vi "James.vi"(0 "Initial Case":enum16{"Theta", "Arc"}(ring), 5 "Drive Case":enum16{"FOD", "ROD"}(ring), 7 "Cyborg":dbl[](array[numeric]), 9 "Logitech":dbl[](array[numeric]), 11 "gyro":dbl format="%#_13g") -> (4 "A":dbl, 6 "B":dbl, 8 "R":dbl)   [LabVIEW 2014]
panel:
  in  "beta":dbl format="%#_13g"
  in  "alpha":dbl format="%#_13g"
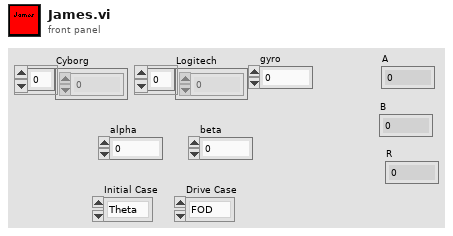
[diagram p1: front panel]
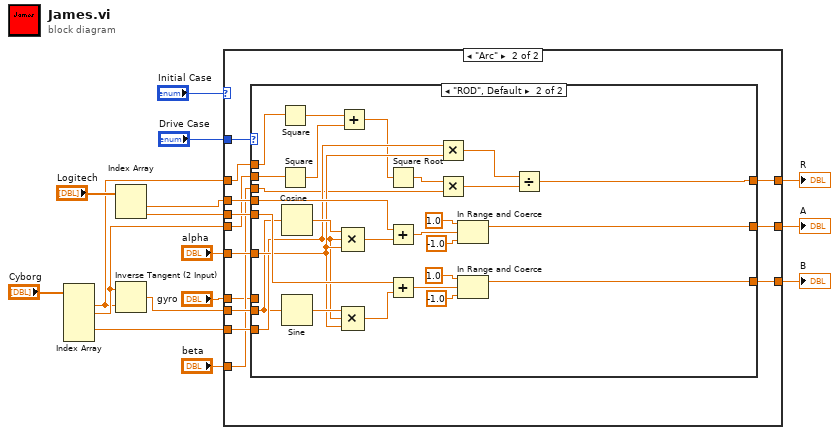
[diagram p0: block diagram]
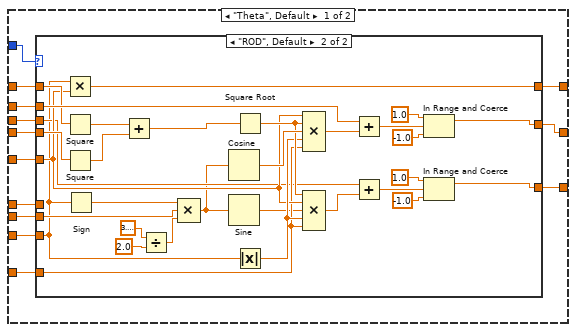
[diagram p2: hidden frame]
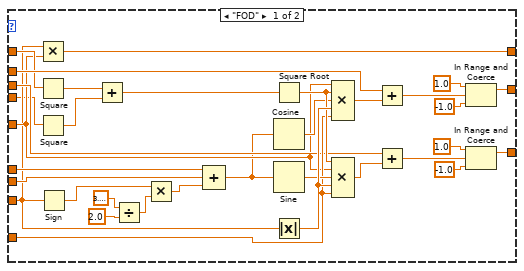
[diagram p3: hidden frame]
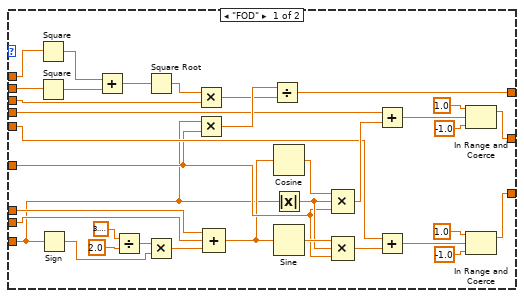
[diagram p4: hidden frame]
diagram:
  n1 = Index Array(array="Cyborg") -> (element #1=w5:dbl, element #2=w6:dbl, element #4=w11:dbl)  [unwired: 5 in, 2 out]
  n2 = Index Array(array="Logitech") -> (element #1=w9:dbl, element #2=w2:dbl)  [unwired: 2 in]
  n3 = Inverse Tangent (2 Input)(1:w5, 2:w6) -> (0:w8:dbl)
  n4 = case shown="\"Arc\"" "Initial Case" {
    tunnel: "Drive Case" -> [w29 w106]
    tunnel: w11 -> [w28 w104]
    tunnel: "alpha" -> [w27 w102]
    tunnel: [w26 w95] -> w13
    tunnel: w9 -> [w25 w105]
    tunnel: w8 -> [w24 w103]
    tunnel: "beta" -> [w23 w98]
    tunnel: w6 -> [w22 w96]
    tunnel: w5 -> [w21 w97]
    tunnel: [w20 w101] -> w4
    tunnel: [w19 w99] -> w3
    tunnel: w2 -> [w18 w100]
    tunnel: "gyro" -> [w17 w94]
    frame "Theta", Default {
      n5 = case shown="\"ROD\", Default" w29 {
        tunnel: w28 -> [w40 w72]
        tunnel: w27 -> [w49 w81]
        tunnel: [w37 w93] -> w26
        tunnel: w25 -> [w52 w92]
        tunnel: w24 -> [w43 w74]
        tunnel: w23 -> [w53 w80]
        tunnel: w22 -> [w39 w89]
        tunnel: w21 -> [w50 w88]
        tunnel: [w34 w64] -> w20
        tunnel: [w30 w69] -> w19
        tunnel: w18 -> [w51 w79]
        tunnel: w17 -> [w41 _]
        frame "FOD" {
          n6 = Multiply(x=w40, y=w49) -> (x*y=w37:dbl)
          n7 = Square(x=w50) -> (x^2=w57:dbl)
          n8 = Square(x=w39) -> (x^2=w56:dbl)
          n9 = Sign(1:w40) -> (0:w48:dbl)
          n10 = Add(x=w57, y=w56) -> (x+y=w58:dbl)
          n11 = Divide(x=3.141592653589793, y=2.0) -> (x/y=w45:dbl)
          n12 = Multiply(x=w48, y=w45) -> (x*y=w44:dbl)
          n13 = Compound Arithmetic op=ADD(w41, w43, w44) -> (w42:dbl)
          n14 = Square Root(x=w58) -> (sqrt(x)=w61:dbl)
          n15 = Cosine(x=w42) -> (cos(x)=w54:dbl)
          n16 = Sine(x=w42) -> (sin(x)=w59:dbl)
          n17 = Absolute Value(x=w40) -> (abs(x)=w62:dbl)
          n18 = Compound Arithmetic op=MULTIPLY(w49, w61, w54, w62, w53) -> (w55:dbl)
          n19 = Compound Arithmetic op=MULTIPLY(w61, w49, w59, w62, w53) -> (w60:dbl)
          n20 = Add(x=w52, y=w55) -> (x+y=w35:dbl)
          n21 = Add(x=w51, y=w60) -> (x+y=w31:dbl)
          n22 = In Range and Coerce(upper limit=1.0, x=w35, lower limit=-1.0) -> (coerced(x)=w34:dbl)  [unwired: 1 out]
          n23 = In Range and Coerce(upper limit=1.0, x=w31, lower limit=-1.0) -> (coerced(x)=w30:dbl)  [unwired: 1 out]
        }
        frame "ROD", Default {
          n24 = Multiply(x=w72, y=w81) -> (x*y=w93:dbl)
          n25 = Square(x=w88) -> (x^2=w86:dbl)
          n26 = Square(x=w89) -> (x^2=w87:dbl)
          n27 = Sign(1:w72) -> (0:w73:dbl)
          n28 = Add(x=w86, y=w87) -> (x+y=w85:dbl)
          n29 = Divide(x=3.141592653589793, y=2.0) -> (x/y=w77:dbl)
          n30 = Compound Arithmetic op=MULTIPLY(w73, w74, w77) -> (w71:dbl)
          n31 = Cosine(x=w71) -> (cos(x)=w91:dbl)
          n32 = Sine(x=w71) -> (sin(x)=w78:dbl)
          n33 = Square Root(x=w85) -> (sqrt(x)=w83:dbl)
          n34 = Absolute Value(x=w72) -> (abs(x)=w82:dbl)
          n35 = Compound Arithmetic op=MULTIPLY(w81, w83, w91, w82, w80) -> (w90:dbl)
          n36 = Compound Arithmetic op=MULTIPLY(w83, w81, w78, w82, w80) -> (w84:dbl)
          n37 = Add(x=w92, y=w90) -> (x+y=w65:dbl)
          n38 = Add(x=w79, y=w84) -> (x+y=w70:dbl)
          n39 = In Range and Coerce(upper limit=1.0, x=w65, lower limit=-1.0) -> (coerced(x)=w64:dbl)  [unwired: 1 out]
          n40 = In Range and Coerce(upper limit=1.0, x=w70, lower limit=-1.0) -> (coerced(x)=w69:dbl)  [unwired: 1 out]
        }
      }
    }
    frame "Arc" {
      n41 = case shown="\"ROD\", Default" w106 {
        tunnel: w105 -> [w130 w168]
        tunnel: w104 -> [w120 w160]
        tunnel: w103 -> [w122 w153]
        tunnel: w102 -> [w125 w161]
        tunnel: [w111 w142] -> w101
        tunnel: w100 -> [w129 w163]
        tunnel: [w107 w146] -> w99
        tunnel: w98 -> [w115 w159]
        tunnel: w97 -> [w128 w156]
        tunnel: w96 -> [w127 w154]
        tunnel: [w131 w151] -> w95
        tunnel: w94 -> [w124 _]
        frame "FOD" {
          n42 = Square(x=w128) -> (x^2=w135:dbl)
          n43 = Square(x=w127) -> (x^2=w134:dbl)
          n44 = Sign(1:w120) -> (0:w121:dbl)
          n45 = Add(x=w135, y=w134) -> (x+y=w132:dbl)
          n46 = Divide(x=3.141592653589793, y=2.0) -> (x/y=w117:dbl)
          n47 = Square Root(x=w132) -> (sqrt(x)=w136:dbl)
          n48 = Multiply(x=w117, y=w121) -> (x*y=w116:dbl)
          n49 = Multiply(x=w136, y=w115) -> (x*y=w133:dbl)
          n50 = Multiply(x=w120, y=w125) -> (x*y=w137:dbl)
          n51 = Compound Arithmetic op=ADD(w124, w122, w116) -> (w123:dbl)
          n52 = Divide(x=w137, y=w133) -> (x/y=w131:dbl)
          n53 = Cosine(x=w123) -> (cos(x)=w140:dbl)
          n54 = Absolute Value(x=w120) -> (abs(x)=w126:dbl)
          n55 = Sine(x=w123) -> (sin(x)=w139:dbl)
          n56 = Compound Arithmetic op=MULTIPLY(w140, w126, w125) -> (w141:dbl)
          n57 = Compound Arithmetic op=MULTIPLY(w139, w126, w125) -> (w138:dbl)
          n58 = Add(x=w130, y=w141) -> (x+y=w112:dbl)
          n59 = Add(x=w129, y=w138) -> (x+y=w108:dbl)
          n60 = In Range and Coerce(upper limit=1.0, x=w112, lower limit=-1.0) -> (coerced(x)=w111:dbl)  [unwired: 1 out]
          n61 = In Range and Coerce(upper limit=1.0, x=w108, lower limit=-1.0) -> (coerced(x)=w107:dbl)  [unwired: 1 out]
        }
        frame "ROD", Default {
          n62 = Square(x=w156) -> (x^2=w157:dbl)
          n63 = Square(x=w154) -> (x^2=w155:dbl)
          n64 = Cosine(x=w153) -> (cos(x)=w166:dbl)
          n65 = Sine(x=w153) -> (sin(x)=w165:dbl)
          n66 = Add(x=w157, y=w155) -> (x+y=w150:dbl)
          n67 = Compound Arithmetic op=MULTIPLY(w166, w160, w161) -> (w167:dbl)
          n68 = Compound Arithmetic op=MULTIPLY(w165, w160, w161) -> (w164:dbl)
          n69 = Square Root(x=w150) -> (sqrt(x)=w158:dbl)
          n70 = Add(x=w168, y=w167) -> (x+y=w143:dbl)
          n71 = Add(x=w163, y=w164) -> (x+y=w147:dbl)
          n72 = Multiply(x=w160, y=w161) -> (x*y=w162:dbl)
          n73 = Multiply(x=w158, y=w159) -> (x*y=w152:dbl)
          n74 = In Range and Coerce(upper limit=1.0, x=w143, lower limit=-1.0) -> (coerced(x)=w142:dbl)  [unwired: 1 out]
          n75 = In Range and Coerce(upper limit=1.0, x=w147, lower limit=-1.0) -> (coerced(x)=w146:dbl)  [unwired: 1 out]
          n76 = Divide(x=w162, y=w152) -> (x/y=w151:dbl)
        }
      }
    }
  }
  "R" <- w13
  "A" <- w4
  "B" <- w3
